vi "Page_Service_Config_Initialize.vi"(6 "ctl references":T1, 8 "error in (no error)":errorcluster, 11 "AB_RESTfulWebService in":refnum<class "AB_RESTfulWebService.lvclass">) -> (0 "error out":errorcluster, 3 "AB_RESTfulWebService out":refnum<class "AB_RESTfulWebService.lvclass">)   [LabVIEW 2020, in "AB_RESTfulWebService.lvclass"]
uses:
  <vilib>/AppBuilder/AB_Classes/RESTful/AB_RESTfulWebService.lvclass
  e:/builds/penguin/labview/branches/2020/dev/dist/vi.lib/AppBuilder/AB_Classes/Build/AB_Build.lvclass
  <resource>/Framework/Providers/Builds/AppBuilder/AB_UI_Page_Service_Config_References.ctl
  <vilib>/AppBuilder/AB_Classes/Build/AB_Build.lvclass
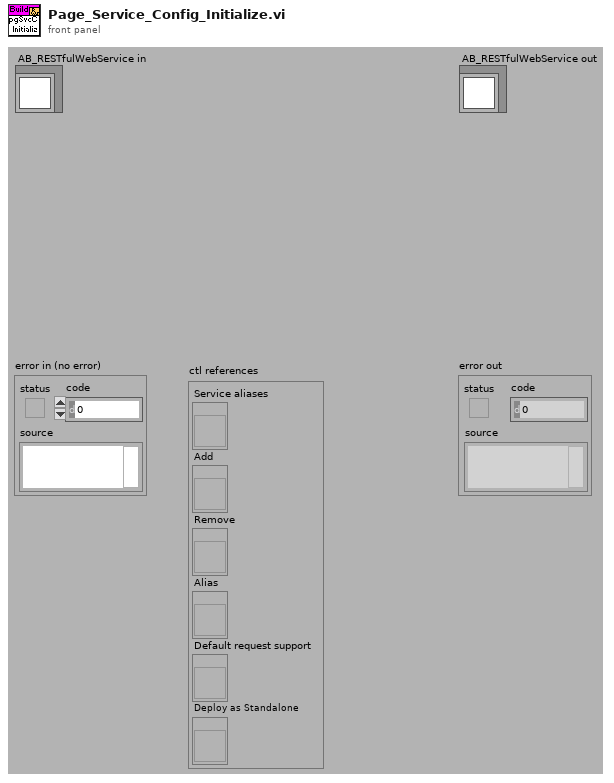
[diagram p1: front panel]
types:
  T1 = typedef "AB_UI_Page_Service_Config_References.ctl" = cluster{"Service aliases":refnum<vi>, "Add":refnum<vi>, "Remove":refnum<vi>, "Alias":refnum<vi>, "Default request support":refnum<vi>, "Deploy as Standalone":refnum<vi>}
  T2 = typedef "AB_Build.ctl" = cluster{"buildSpecName":string, "buildSpecDescription":string, "destinations":refnum<class "AB_Destination.lvclass">[], "exclusionOption":T3, "defaultLanguage":string, "supportedLanguages":string[], "excludedDirectories":path[], "buildContext":refnum<vi>, "buildObject":T4, "preview":bool, "programatic":bool, "progressBarEvents":T5, "userLog_Path":path, "preActionID":string, "preAction_Path":path, "postActionID":string, "postAction_Path":path, "eng_checkForBrokenVIs?":bool, "eng_verboseLinkerErrors?":bool, "localDest_Path":path, "targetDest_Path":path, "removeVIObject":u16, "cache":refnum<class "PreviewCache.lvclass">, "use cache":bool, "previewCache_ID":string, "buildCache_ID":string, "eng_TempLocalDest_Path":path, "eng_collectDependencies?":bool, "versionInfo":cluster{"buildVersion":cluster{"major":u16, "minor":u16, "patch":u16, "build":u16}, "autoIncrement":bool}, "eng_enableVIChecksums":bool}
  T3 = typedef "AB_Exclusion_Option.ctl" = cluster{"typedefs":bool, "polymorphicVIs":bool, "unusedLibraryItems":bool, "modifyLibraryFile":bool, "edit-timeDependencies":bool, "inlineVIs":bool, "dependent PPLs":bool, "dependent DLLs":bool}
  T4 = typedef "ItemRef.ctl" = u64
  T5 = typedef "provcom_ProgressBar_Events.ctl" = cluster{"newJob":refnum<user-event>, "newItem":refnum<user-event>, "errorMsg":T6, "cancel":refnum<user-event>}
  T6 = typedef "mxLvBuildError.ctl" = refnum<user-event>
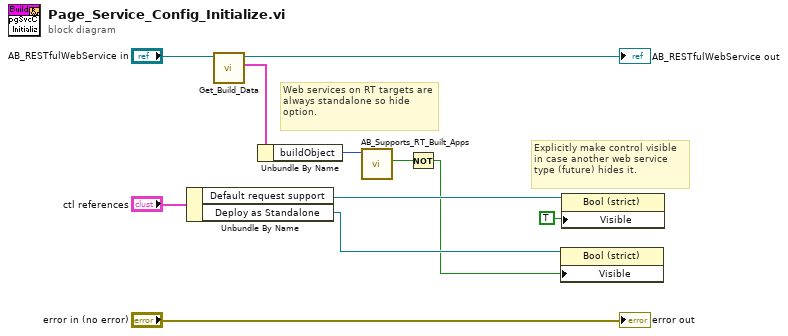
[diagram p0: block diagram]
diagram:
  # "Web services on RT targets are always standalone so hide option."
  # "Explicitly make control visible in case another web service type (future) hides it."
  n1 = Unbundle By Name("ctl references") -> ("Default request support"=w8:refnum<vi>, "Deploy as Standalone"=w3:refnum<vi>)
  n2 = call <vilib>:"Get_Build_Data.vi"("Class in"="AB_RESTfulWebService in") -> ("data"=w5:T2, "Class out"=→"AB_RESTfulWebService out":refnum<class "AB_RESTfulWebService.lvclass">)  [unwired: 8 in, 1 out]
  n3 = Unbundle By Name(w5) -> ("buildObject"=w4:T4)
  n4 = call <resource>:"AB_Supports_RT_Built_Apps.vi"("Object"=w4) -> ("SupportsRTBuiltApps"=w2:bool)  [unwired: 8 in, 2 out]
  n5 = Not(x=w2) -> (.not. x?=w1:bool)
  n6 = property class="Bool (strict)"(reference=w3, "Visible"=w1) -> ()  [unwired: 1 in, 2 out]
  n7 = property class="Bool (strict)"(reference=w8, "Visible"=TRUE) -> ()  [unwired: 1 in, 2 out]
  "error out" <- "error in (no error)"
